vi "fornum.vi"() -> ()   [LabVIEW 2022 SP3]
panel:
  out "数组":i32[](array[numeric])
  out "大小":i32=10
  out "结果字符串":string="9"
  out "Number":i32=9
  out "x+y":i32=300
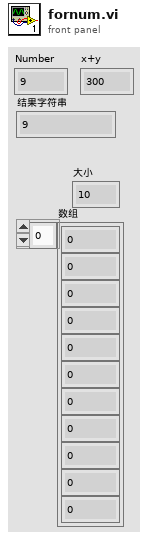
[diagram p1: front panel]
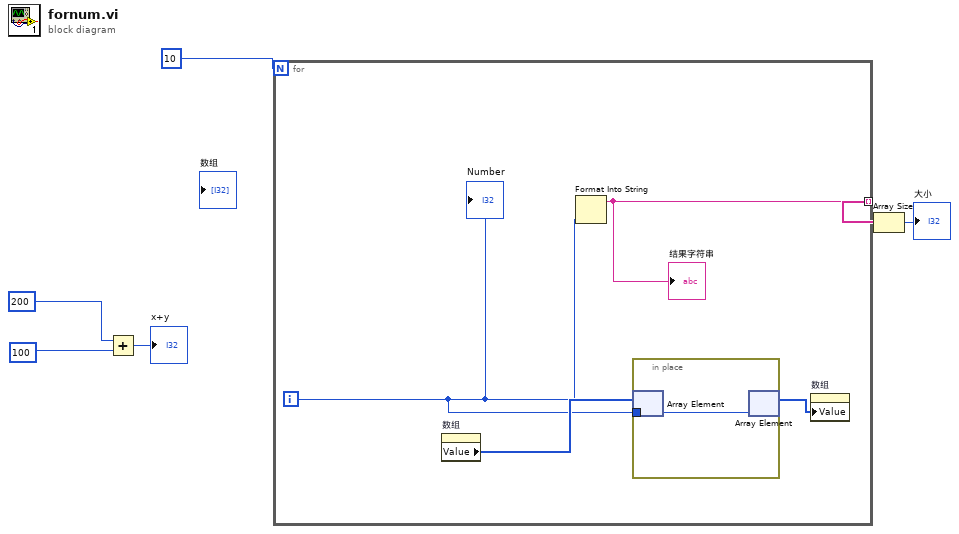
[diagram p0: block diagram]
diagram:
  n1 = Add(x=200, y=100) -> (x+y=→"x+y":i32)
  n2 = for {
    N: 10 -> [_]
    tunnel: [w10] -> w2 mode=indexing
    i -> [w8]
    n3 = property on="数组" class="Arr (严格)"() -> ("Value"=w9:i32[])  [unwired: 2 in, 2 out]
    n4 = Format Into String(w8) -> (resulting string=w10:string)  [unwired: 3 in, 1 out]
    "结果字符串" <- w10
    n5 = in-place {
      in-place-border: w8 -> [w11]
      n6 = in-place-array #1(w9, w8) -> ()  [unwired: 1 out]
      n7 = in-place-array #1(w11) -> (w7:i32[])  [unwired: 1 out]
    }
    n8 = property on="数组" class="Arr (严格)"("Value"=w7) -> ()  [unwired: 2 in, 2 out]
    "Number" <- w8
  }
  n9 = Array Size(array=w2) -> (size(s)=→"大小":i32)
